vi "Trajectory Loading v2.vi"(6 "PID Cluster":T5={"L1 to L4 PID Cluster"={"L1 PID Gains"={"Kp"=0.005, "Kd"=0.5, "Ki"=0.0005}, "L2 PID Gains"={"Kp"=0.01, "Kd"=1.0, "Ki"=0.005}, "L3 PID Gains"={"Kp"=0.05, "Kd"=1.0, "Ki"=0.0005}, "L4 PID Gains"={"Kp"=0.1, "Kd"=0.1, "Ki"=0.0005}}, "Stage PID Cluster"={"Stage Z PID"={"Kp"=0.0005, "Kd"=0.001, "Ki"=0.0}, "Stage Y PID"={"Kp"=0.0003, "Kd"=0.01, "Ki"=0.0}, "Stage X PID"={"Kp"=0.0003, "Kd"=0.01, "Ki"=0.0}}, "OCT Z PID Gains"={"Kp"=0.0003, "Kd"=0.0001, "Ki"=0.01}}, 8 "error in":errorcluster, 9 "Offset Home 2 RCM":dbl[](array[numeric])=[0.0, 0.0, 0.0, 0.0], 10 "Prev Posit Cluster":T4={"Prev L1 to L4 Posit"=[-0.5319, -0.035669172703475985, -2.0566170657346783, 0.9099264705882353], "Prev Stage Posit"=[6.002553885707208, 5.996566124542428, 5.995469940427586], "Prev OCT Z Posit"=-0.0}, 11 "FPGA VI Reference In":refnum<k20>) -> (0 "RUY Cluster":T1, 1 "Trajectory Cluster":T2, 2 "Last Posit Cluster":T3={"Last L1 to L4 Posit"=[0.0, 0.0, 0.0, 0.0], "Last Stage Posit"=[6.0, 6.0, 6.0], "Last OCT Z Posit"=0.0}, 3 "FPGA VI Reference Out":refnum<k20>, 4 "error out":errorcluster, 5 "First Trk Pt":dbl[](array[numeric]))   [LabVIEW 2016]
uses:
  <vilib>/Platform/TimedLoop/XDataNode/timing_clust.ctl
  <vilib>/Platform/TimedLoop/XDataNode/nitl_modes.ctl
  <vilib>/Platform/TimedLoop/XDataNode/wakeup.ctl
  Global Variables.vi
  <vilib>/platform/TimedLoop/XDataNode/XDataNode.xnode
  <vilib>/Platform/TimedLoop/XDataNode/XDNodeRunTimeDep.lvlib
panel:
  out "In Servo Loop":bool
  out "Loading Finished":bool
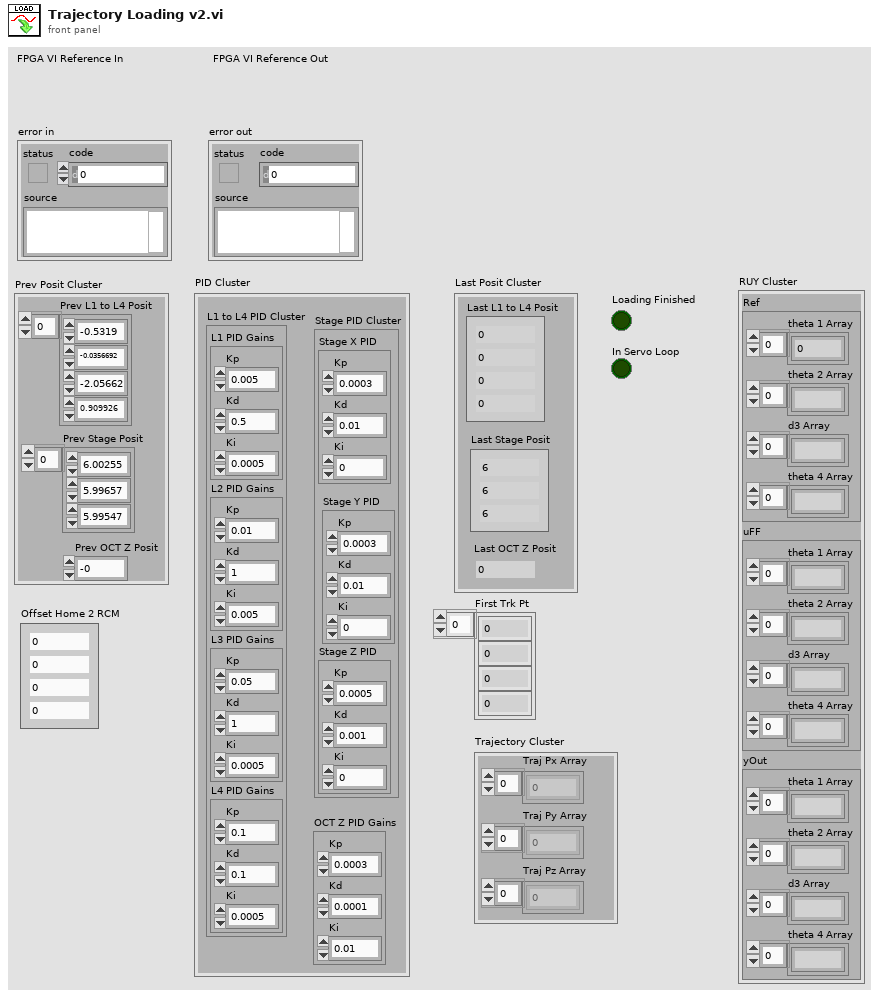
[diagram p1: front panel]
types:
  T1 = cluster{"Ref":cluster{"theta 1 Array":dbl[], "theta 2 Array":dbl[], "d3 Array":dbl[], "theta 4 Array":dbl[]}, "uFF":cluster{"theta 1 Array":dbl[], "theta 2 Array":dbl[], "d3 Array":dbl[], "theta 4 Array":dbl[]}, "yOut":cluster{"theta 1 Array":dbl[], "theta 2 Array":dbl[], "d3 Array":dbl[], "theta 4 Array":dbl[]}}
  T2 = cluster{"Traj Px Array":dbl[], "Traj Py Array":dbl[], "Traj Pz Array":dbl[]}
  T3 = cluster{"Last L1 to L4 Posit":dbl[], "Last Stage Posit":dbl[], "Last OCT Z Posit":dbl}
  T4 = cluster{"Prev L1 to L4 Posit":dbl[], "Prev Stage Posit":dbl[], "Prev OCT Z Posit":dbl}
  T5 = cluster{"L1 to L4 PID Cluster":cluster{"L1 PID Gains":cluster{"Kp":dbl, "Kd":dbl, "Ki":dbl}, "L2 PID Gains":cluster{"Kp":dbl, "Kd":dbl, "Ki":dbl}, "L3 PID Gains":cluster{"Kp":dbl, "Kd":dbl, "Ki":dbl}, "L4 PID Gains":cluster{"Kp":dbl, "Kd":dbl, "Ki":dbl}}, "Stage PID Cluster":cluster{"Stage Z PID":cluster{"Kp":dbl, "Kd":dbl, "Ki":dbl}, "Stage Y PID":cluster{"Kp":dbl, "Kd":dbl, "Ki":dbl}, "Stage X PID":cluster{"Kp":dbl, "Kd":dbl, "Ki":dbl}}, "OCT Z PID Gains":cluster{"Kp":dbl, "Kd":dbl, "Ki":dbl}}
  T6 = typedef "XDNodeRunTimeDep.lvlib/timing_clust.ctl" = cluster{"Expected End [f-1]":u64, "Actual End [f-1]":u64, "Finished Late? [f-1]":bool, "Expected End [i-1]":u64, "Actual End [i-1]":u64, "Finished Late? [i-1]":bool, "Expected Start [i]":u64, "Actual Start [i]":u64, "Expected Start [f]":u64, "Actual Start [f]":u64, "Source Name":string, "Structure Name":string, "Period":i64, "Deadline":i64, "Offset":i64, "Start":i64, "Priority":i32, "Timeout":i32, "Mode":T7, "Wakeup Reason":T8, "Error":errorcluster, "Source Type":string, "Secondary Source Type":string, "Global End Time":u64, "Global Start Time":u64, "Frame Duration":u64, "Iteration Duration":u64, "Assigned CPU":i32, "I/O Scan Engine Mode":u32}
  T7 = typedef "XDNodeRunTimeDep.lvlib/nitl_modes.ctl" = enum32{"No Change", "Process missed periods, maintain original phase", "Discard missed periods, maintain original phase", "Process missed periods, ignore original phase", "Discard missed periods, ignore original phase"}
  T8 = typedef "XDNodeRunTimeDep.lvlib/wakeup.ctl" = enum32{"Normal", "Aborted", "Asynchronous wakeup", "Timing source error", "Timed loop error", "Timeout"}
  T9 = cluster{"theta 1 Array":dbl[], "theta 2 Array":dbl[], "d3 Array":dbl[], "theta 4 Array":dbl[]}
  T10 = cluster{"L1 PID Gains":cluster{"Kp":dbl, "Kd":dbl, "Ki":dbl}, "L2 PID Gains":cluster{"Kp":dbl, "Kd":dbl, "Ki":dbl}, "L3 PID Gains":cluster{"Kp":dbl, "Kd":dbl, "Ki":dbl}, "L4 PID Gains":cluster{"Kp":dbl, "Kd":dbl, "Ki":dbl}}
  T11 = cluster{"Stage Z PID":cluster{"Kp":dbl, "Kd":dbl, "Ki":dbl}, "Stage Y PID":cluster{"Kp":dbl, "Kd":dbl, "Ki":dbl}, "Stage X PID":cluster{"Kp":dbl, "Kd":dbl, "Ki":dbl}}
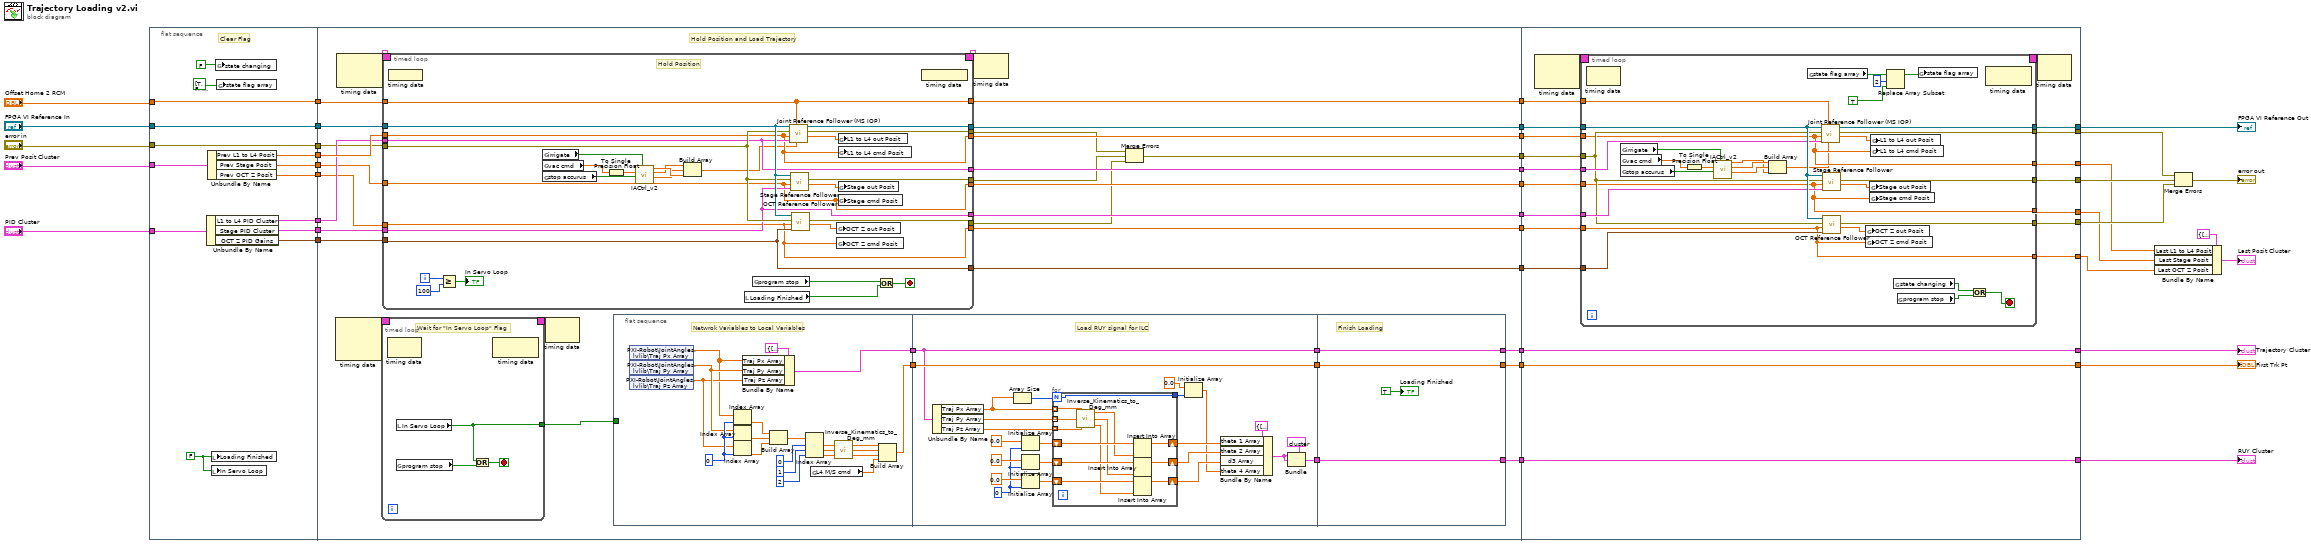
[diagram p0: block diagram]
diagram:
  n1 = flat-sequence {
    tunnel: [w51] -> w39
    tunnel: "FPGA VI Reference In" -> [w51]
    tunnel: [w50] -> w37
    tunnel: "error in" -> [w50]
    tunnel: "Prev Posit Cluster" -> [w49]
    tunnel: "PID Cluster" -> [w48]
    tunnel: [w47] -> w35
    tunnel: [w46] -> w34
    tunnel: "Offset Home 2 RCM" -> [w45]
    tunnel: [w45] -> w32
    tunnel: [w44] -> w29
    tunnel: [w43] -> w28
    tunnel: [w42] -> w27
    tunnel: [w41] -> w26
    tunnel: w39 -> [w73]
    tunnel: w37 -> [w68]
    tunnel: w35 -> [w70]
    tunnel: w34 -> [w69]
    tunnel: w32 -> [w74]
    tunnel: w29 -> [w72]
    tunnel: w28 -> [w67]
    tunnel: w27 -> [w66]
    tunnel: w26 -> [w71]
    tunnel: [w87] -> w14
    tunnel: [w86] -> w13
    tunnel: [w85] -> w12
    tunnel: [w84] -> w11
    tunnel: [w83] -> w10
    tunnel: [w82] -> w9
    tunnel: [w81] -> w8
    tunnel: [w80] -> w7
    tunnel: [w62] -> w6
    tunnel: [w61] -> w5
    tunnel: [w60] -> w4
    tunnel: [w54] -> w2
    tunnel: w14 -> [w208]
    tunnel: [w207] -> w24
    tunnel: [w206] -> w23
    tunnel: [w205] -> w22
    tunnel: w13 -> [w204]
    tunnel: w12 -> [w203]
    tunnel: w11 -> [w202]
    tunnel: w10 -> [w201]
    tunnel: w9 -> [w200]
    tunnel: w8 -> [w199]
    tunnel: w7 -> [w198]
    tunnel: [w197] -> w20
    tunnel: [w196] -> w19
    tunnel: [w195] -> w18
    tunnel: [w194] -> w16
    tunnel: [w191] -> w15
    tunnel: w6 -> [w193]
    tunnel: w5 -> [w191]
    tunnel: [w192] -> w3
    tunnel: w4 -> [w192]
    tunnel: w2 -> [w190]
    tunnel: [w190] -> w1
    frame #0 {
      w40 = FALSE ("Loading Finished")
      # "Clear Flag"
      n2 = Unbundle By Name(w48) -> ("L1 to L4 PID Cluster"=w46:T10, "Stage PID Cluster"=w47:T11, "OCT Z PID Gains"=w41:cluster{"Kp":dbl, "Kd":dbl, "Ki":dbl})
      n3 = Unbundle By Name(w49) -> ("Prev L1 to L4 Posit"=w44:dbl[], "Prev Stage Posit"=w43:dbl[], "Prev OCT Z Posit"=w42:dbl)
      n4 = local write "Loading Finished"(w40) -> ()
      n5 = local write "In Servo Loop"(w40) -> ()
      n6 = global write "Global Variables.vi" "state changing"(FALSE ("state changing")) -> ()
      n7 = global write "Global Variables.vi" "state flag array"(bool[] [TRUE, FALSE, FALSE, FALSE, FALSE, FALSE, FALSE, FALSE, FALSE] ("state flag array")) -> ()
    }
    frame #1 {
      # "Hold Position and Load Trajectory"
      n8 = node-c288() -> (w77:T6)  [unwired: 3 in]
      n9 = node-c288() -> (w79:T6)  [unwired: 2 in]
      n10 = timed-loop {
        timing: w77 -> [_]
        timing-out: [_] -> w76
        tunnel: [w89] -> w75
        stop <- w90 stop-if-true
        # "Wait for \"In Servo Loop\" Flag"
        n11 = node-c288() -> ()  [unwired: 1 in, 1 out]
        n12 = local read "In Servo Loop"() -> (w89:bool)
        n13 = global read "Global Variables.vi" "program stop"() -> (w88:bool)
        n14 = Or(x=w89, y=w88) -> (x .or. y?=w90:bool)
        n15 = node-c288() -> ()  [unwired: 1 in, 1 out]
      }
      n16 = timed-loop {
        timing: w79 -> [_]
        timing-out: [_] -> w78
        tunnel: w72 -> [w166]
        tunnel: w67 -> [w165]
        tunnel: w70 -> [w170]
        tunnel: w69 -> [w171]
        tunnel: w68 -> [w181]
        tunnel: w73 -> [w182]
        tunnel: w74 -> [w177]
        tunnel: w66 -> [w164]
        tunnel: w71 -> [w172]
        tunnel: [w166] -> w85
        tunnel: [w165] -> w84
        tunnel: [w164] -> w83
        tunnel: [w177] -> w86
        tunnel: [w176] -> w87
        tunnel: [w175] -> w65
        tunnel: [w174] -> w64
        tunnel: [w173] -> w63
        tunnel: [w172] -> w82
        tunnel: [w171] -> w81
        tunnel: [w170] -> w80
        i -> [w169]
        stop <- w185 stop-if-true
        # "Hold Position"
        n17 = node-c288 ("Output Node")() -> ()  [unwired: 1 in]
        n18 = Greater Or Equal?(x=w169, y=100) -> (x >= y?=→"In Servo Loop":bool)
        n19 = global read "Global Variables.vi" "irrigate"() -> (w162:bool)
        n20 = global read "Global Variables.vi" "vac cmd"() -> (w156:sgl)
        n21 = global read "Global Variables.vi" "stop accurus"() -> (w158:bool)
        n22 = To Single Precision Float(number=w156) -> (single precision float=w157:sgl)
        n23 = call "IACtrl_v2.vi"("Irrigate?"=w162, "E-Stop Vacuum"=w158, "Vacuum Force [mmHg]"=w157) -> ("Accurus ChB Vout"=w160:dbl, "Accurus ChA Vout"=w161:dbl, "Accurus Engaged Vout"=w163:dbl)  [unwired: 5 in, 1 out]
        n24 = Build Array(w161, w160, w163) -> (w159:dbl[])
        n25 = local read "Loading Finished"() -> (w184:bool)
        n26 = global read "Global Variables.vi" "program stop"() -> (w183:bool)
        n27 = call "Joint Reference Follower (MS IOP).vi"("Acc Ctrl Array"=w159, "Offset Home2RCM [deg/mm]"=w177, "PID Ctrl Cluster"=w171, "Ref Array [deg/mm]"=w166, "error in"=w181, "FPGA VI Reference In"=w182) -> ("Output Posit Array [deg/mm]"=w180:dbl[], "error out"=w175:errorcluster, "FPGA VI Reference Out"=w176:refnum<k20>)  [unwired: 3 in]
        n28 = call "Stage Reference Follower.vi"("Stage PID Cluster"=w170, "Stage cmd Posit [mm]"=w165, "error in"=w181, "FPGA VI Reference In"=w182) -> ("Stage out Posit [mm]"=w179:dbl[], "error out"=w174:errorcluster)  [unwired: 5 in, 1 out]
        n29 = call "OCT Reference Follower.vi"("OCT Z PID Gains"=w172, "OCT  Z cmd Posit [mm]"=w164, "error in"=w181, "FPGA VI Reference In"=w182) -> ("OCT  Z out Posit [mm]"=w178:dbl, "error out"=w173:errorcluster)  [unwired: 5 in, 1 out]
        n30 = global write "Global Variables.vi" "OCT Z out Posit"(w178) -> ()
        n31 = global write "Global Variables.vi" "OCT Z cmd Posit"(w164) -> ()
        n32 = global write "Global Variables.vi" "L1 to L4 out Posit"(w180) -> ()
        n33 = global write "Global Variables.vi" "L1 to L4 cmd Posit"(w166) -> ()
        n34 = global write "Global Variables.vi" "Stage out Posit"(w179) -> ()
        n35 = global write "Global Variables.vi" "Stage cmd Posit"(w165) -> ()
        n36 = Or(x=w183, y=w184) -> (x .or. y?=w185:bool)
        n37 = node-c288() -> ()  [unwired: 1 out]
      }
      n38 = node-c288(w76) -> ()  [unwired: 1 out]
      n39 = flat-sequence {
        tunnel: [w114] -> w59
        tunnel: w75 -> [_]
        tunnel: [w97] -> w57
        tunnel: w59 -> [w126]
        tunnel: [w126] -> w58
        tunnel: w57 -> [w138]
        tunnel: [w138] -> w56
        tunnel: [w120] -> w55
        tunnel: w58 -> [w154]
        tunnel: [w154] -> w61
        tunnel: [w153] -> w60
        tunnel: w56 -> [w153]
        tunnel: w55 -> [w152]
        tunnel: [w152] -> w54
        frame #0 {
          w112 = 0 ("index")
          # "Netwrok Variables to Local Variables"
          n40 = shared-variable "PXI-Robot\\JointAngles.lvlib\\Traj Px Array"() -> (w95:dbl[])  [unwired: 1 in, 1 out]
          n41 = shared-variable "PXI-Robot\\JointAngles.lvlib\\Traj Py Array"() -> (w99:dbl[])  [unwired: 1 in, 1 out]
          n42 = shared-variable "PXI-Robot\\JointAngles.lvlib\\Traj Pz Array"() -> (w98:dbl[])  [unwired: 1 in, 1 out]
          n43 = Index Array(array=w95, index=w112) -> (element=w100:dbl)
          n44 = Index Array(array=w99, index=w112) -> (element=w101:dbl)
          n45 = Index Array(array=w98, index=w112) -> (element=w102:dbl)
          n46 = Bundle By Name(cluster=T2 {"Traj Px Array"=[], "Traj Py Array"=[], "Traj Pz Array"=[]} ("Trajectory Cluster"), "Traj Px Array"=w95, "Traj Py Array"=w99, "Traj Pz Array"=w98) -> (w114:T2)
          n47 = Build Array(w100, w101, w102) -> (w113:dbl[])
          n48 = Index Array(array=w113, index #1=0 ("index"), index #2=1 ("index"), index #3=2 ("index")) -> (element #1=w107:dbl, element #2=w109:dbl, element #3=w108:dbl)
          n49 = global read "Global Variables.vi" "L4 M/S cmd"() -> (w96:dbl)
          n50 = call "Inverse_Kinematics_to_Deg_mm.vi"("pz"=w108, "py"=w109, "px"=w107) -> ("L3 [mm]"=w104:dbl, "L2 [deg]"=w105:dbl, "L1 [deg]"=w106:dbl)
          n51 = Build Array(w106, w105, w104, w96) -> (w97:dbl[])
        }
        frame #1 {
          w130 = 0 ("dimension size")
          # "Load RUY signal for ILC"
          n52 = Unbundle By Name(w126) -> ("Traj Px Array"=w136:dbl[], "Traj Py Array"=w134:dbl[], "Traj Pz Array"=w135:dbl[])
          n53 = Array Size(array=w136) -> (size(s)=w137:i32)
          n54 = Initialize Array(0.0 ("element"), w130) -> (w129:dbl[])
          n55 = Initialize Array(0.0 ("element"), w130) -> (w128:dbl[])
          n56 = Initialize Array(0.0 ("element"), w130) -> (w127:dbl[])
          n57 = for {
            N: w137 -> [w139]
            tunnel: w136 -> [w151] mode=indexing
            tunnel: w135 -> [w150] mode=indexing
            tunnel: w134 -> [w149] mode=indexing
            shift-right: [w142] -> w119
            shift-left: w129 -> [w148]
            shift-right: [w141] -> w117
            shift-left: w128 -> [w146]
            shift-right: [w140] -> w118
            shift-left: w127 -> [w144]
            tunnel: [w139] -> w123
            n58 = call "Inverse_Kinematics_to_Deg_mm.vi"("pz"=w150, "py"=w149, "px"=w151) -> ("L3 [mm]"=w143:dbl, "L2 [deg]"=w145:dbl, "L1 [deg]"=w147:dbl)
            n59 = Insert Into Array(array=w148, new element=w147) -> (w142:dbl[])  [unwired: 1 in]
            n60 = Insert Into Array(array=w146, new element=w145) -> (w141:dbl[])  [unwired: 1 in]
            n61 = Insert Into Array(array=w144, new element=w143) -> (w140:dbl[])  [unwired: 1 in]
          }
          n62 = Initialize Array(0.0 ("element"), w123) -> (w116:dbl[])
          n63 = Bundle By Name(cluster=T9 {"theta 1 Array"=[], "theta 2 Array"=[], "d3 Array"=[], "theta 4 Array"=[]} ("uFF"), "theta 1 Array"=w119, "theta 2 Array"=w117, "d3 Array"=w118, "theta 4 Array"=w116) -> (w121:T9)
          n64 = Bundle(cluster=T1 {"Ref"={"theta 1 Array"=array[6000 elements], "theta 2 Array"=array[6000 elements], "d3 Array"=array[6000 elements], "theta 4 Array"=array[6000 elements]}, "uFF"={"theta 1 Array"=array[6000 elements], "theta 2 Array"=array[6000 elements], "d3 Array"=array[6000 elements], "theta 4 Array"=array[6000 elements]}, "yOut"={"theta 1 Array"=[], "theta 2 Array"=[], "d3 Array"=[], "theta 4 Array"=[]}} ("Cluster"), "Ref"=w121, "uFF"=w121) -> (w120:T1)  [unwired: 1 in]
        }
        frame #2 {
          # "Finish Loading"
          "Loading Finished" <- TRUE ("Loading Finished")
        }
      }
      n65 = node-c288(w78) -> ()  [unwired: 1 out]
      n66 = Merge Errors(w65, w64, w63) -> (w62:errorcluster)
    }
    frame #2 {
      n67 = node-c288() -> (w210:T6)  [unwired: 2 in]
      n68 = timed-loop {
        timing: w210 -> [_]
        timing-out: [_] -> w209
        tunnel: w208 -> [w234]
        tunnel: [w233] -> w206
        tunnel: [w232] -> w207
        tunnel: [w231] -> w205
        tunnel: w204 -> [w230]
        tunnel: w203 -> [w221]
        tunnel: w202 -> [w220]
        tunnel: w201 -> [w219]
        tunnel: w200 -> [w229]
        tunnel: w199 -> [w228]
        tunnel: w198 -> [w227]
        tunnel: [w221] -> w197
        tunnel: [w220] -> w196
        tunnel: [w219] -> w195
        tunnel: [w223] -> w194
        tunnel: w193 -> [w222]
        stop <- w241 stop-if-true
        n69 = node-c288() -> ()  [unwired: 1 in, 1 out]
        n70 = global read "Global Variables.vi" "irrigate"() -> (w213:bool)
        n71 = global read "Global Variables.vi" "vac cmd"() -> (w218:sgl)
        n72 = global read "Global Variables.vi" "stop accurus"() -> (w216:bool)
        n73 = To Single Precision Float(number=w218) -> (single precision float=w217:sgl)
        n74 = call "IACtrl_v2.vi"("Irrigate?"=w213, "E-Stop Vacuum"=w216, "Vacuum Force [mmHg]"=w217) -> ("Accurus ChB Vout"=w215:dbl, "Accurus ChA Vout"=w214:dbl, "Accurus Engaged Vout"=w212:dbl)  [unwired: 5 in, 1 out]
        n75 = Build Array(w214, w215, w212) -> (w211:dbl[])
        n76 = global read "Global Variables.vi" "state flag array"() -> (w238:bool[])
        n77 = call "Joint Reference Follower (MS IOP).vi"("Acc Ctrl Array"=w211, "Offset Home2RCM [deg/mm]"=w230, "PID Ctrl Cluster"=w228, "Ref Array [deg/mm]"=w221, "error in"=w222, "FPGA VI Reference In"=w234) -> ("Output Posit Array [deg/mm]"=w226:dbl[], "error out"=w233:errorcluster, "FPGA VI Reference Out"=w223:refnum<k20>)  [unwired: 3 in]
        n78 = call "Stage Reference Follower.vi"("Stage PID Cluster"=w227, "Stage cmd Posit [mm]"=w220, "error in"=w222, "FPGA VI Reference In"=w234) -> ("Stage out Posit [mm]"=w225:dbl[], "error out"=w232:errorcluster)  [unwired: 5 in, 1 out]
        n79 = call "OCT Reference Follower.vi"("OCT Z PID Gains"=w229, "OCT  Z cmd Posit [mm]"=w219, "error in"=w222, "FPGA VI Reference In"=w234) -> ("OCT  Z out Posit [mm]"=w224:dbl, "error out"=w231:errorcluster)  [unwired: 5 in, 1 out]
        n80 = global write "Global Variables.vi" "OCT Z out Posit"(w224) -> ()
        n81 = global write "Global Variables.vi" "OCT Z cmd Posit"(w219) -> ()
        n82 = global write "Global Variables.vi" "Stage out Posit"(w225) -> ()
        n83 = global write "Global Variables.vi" "Stage cmd Posit"(w220) -> ()
        n84 = global write "Global Variables.vi" "L1 to L4 out Posit"(w226) -> ()
        n85 = global write "Global Variables.vi" "L1 to L4 cmd Posit"(w221) -> ()
        n86 = Replace Array Subset(array=w238, new element=TRUE ("new element/subarray"), index=2) -> (w237:bool[])
        n87 = global read "Global Variables.vi" "state changing"() -> (w240:bool)
        n88 = global read "Global Variables.vi" "program stop"() -> (w239:bool)
        n89 = global write "Global Variables.vi" "state flag array"(w237) -> ()
        n90 = Or(x=w240, y=w239) -> (x .or. y?=w241:bool)
        n91 = node-c288() -> ()  [unwired: 1 in, 1 out]
      }
      n92 = node-c288(w209) -> ()  [unwired: 1 out]
    }
  }
  n93 = Bundle By Name(cluster=T3 {"Last L1 to L4 Posit"=[0.0, 0.0, 0.0, 0.0], "Last Stage Posit"=[6.0, 6.0, 6.0], "Last OCT Z Posit"=0.0} ("Last Posit Cluster 2"), "Last L1 to L4 Posit"=w20, "Last Stage Posit"=w19, "Last OCT Z Posit"=w18) -> (→"Last Posit Cluster":T3)
  n94 = Merge Errors(w23, w24, w22) -> (→"error out":errorcluster)
  "FPGA VI Reference Out" <- w16
  "First Trk Pt" <- w3
  "Trajectory Cluster" <- w15
  "RUY Cluster" <- w1
